vi "Do.vi"(8 "error in (no error)":errorcluster, 10 "Actor in":refnum<class "Actor.lvclass">, 11 "Update_Referenced Msg":refnum<class "Update_Referenced Msg.lvclass">) -> (0 "error out":errorcluster, 2 "Actor out":refnum<class "Actor.lvclass">)   [LabVIEW 2016, in "CS++Motor.lvlib" / "Update_Referenced Msg.lvclass"]
doc: "This VI delivers the message to the actor by calling the appropriate method(s) on the actor."
uses:
  Update_Referenced Msg.lvclass
  <vilib>/ActorFramework/Actor/Actor.lvclass
  C:/User/Brand/LVP/CSPP-Dev/Packages/CSPP_Core/Actors/CS++PVMonitor Messages/CS++PVUpdate Msg/CS++PVUpdate Msg.lvclass
  CS++Motor/CS++Motor.lvclass
  C:/Program Files (x86)/National Instruments/LabVIEW 2016/vi.lib/ActorFramework/Actor/Actor.lvclass
  CSPP_Core/Actors/CS++PVMonitor Messages/CS++PVUpdate Msg/CS++PVUpdate Msg.lvclass/CS++PVUpdate Msg.ctl
  CSPP_Core/Classes/CS++ProcessVariables/ProcessVariable/PV.lvclass/PV.ctl
  CSPP_Core/Classes/CS++ProcessVariables/ProcessVariable/PV.lvclass
  CSPP_Core/Actors/CS++PVMonitor Messages/CS++PVUpdate Msg/CS++PVUpdate Msg.lvclass
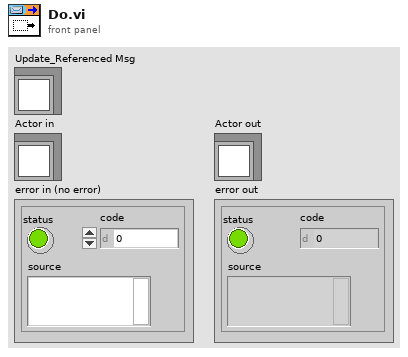
[diagram p1: front panel]
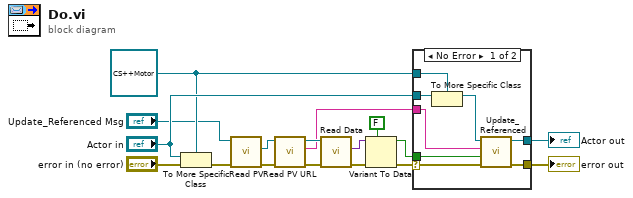
[diagram p0: block diagram]
diagram:
  w13 = refnum<class "CS++Motor.lvclass"> refnum ("Actor in")
  n1 = To More Specific Class(target class=w13, reference="Actor in", error in="error in (no error)") -> (error out=w8:errorcluster)  [unwired: 1 out]
  n2 = call "Read PV.vi"("error in (no error)"=w8, "CS++PVUpdate Msg in"="Update_Referenced Msg") -> ("error out"=w5:errorcluster, "PV"=w3:refnum<class "PV.lvclass">)  [unwired: 7 in, 1 out]
  n3 = call "Read PV URL.vi"("error in (no error)"=w5, "PV in"=w3) -> ("error out"=w4:errorcluster, "PV URL"=w1:string, "PV out"=w2:refnum<class "PV.lvclass">)  [unwired: 7 in]
  n4 = call "Read Data.vi"("error in (no error)"=w4, "PV in"=w2) -> ("error out"=w9:errorcluster, "Data"=w10:variant)  [unwired: 7 in, 1 out]
  n5 = Variant To Data(error in=w9, type=FALSE ("Referenced?"), Variant=w10) -> (data=w6:bool, error out=w7:errorcluster)
  n6 = case shown="No Error" w7 {
    selector: w7 -> [w23 w27]
    tunnel: [w25 w27] -> w16
    tunnel: [w24 w26] -> w15
    tunnel: "Actor in" -> [w22 w26]
    tunnel: w13 -> [w21 _]
    tunnel: w6 -> [w19 _]
    tunnel: w1 -> [w18 _]
    frame No Error {
      n7 = To More Specific Class(target class=w21, reference=w22) -> (specific class reference=w20:refnum<class "CS++Motor.lvclass">)  [unwired: 1 in, 1 out]
      n8 = call "Update_Referenced.vi"("error in (no error)"=w23, "Referenced?"=w19, "PV-URL"=w18, "CS++Motor in"=w20) -> ("error out"=w25:errorcluster, "CS++Motor out"=w24:refnum<class "CS++Motor.lvclass">)  [unwired: 6 in]
    }
    frame Error {
    }
  }
  "error out" <- w16
  "Actor out" <- w15
